vi "Create from Cluster.vi"(7 "Write Lock":refnum<notifier>, 8 "error in (no error)":errorcluster, 10 "Ref Data":T1={"Node Info"={"Index"=-1, "Parent"=-1, "Children"=[]}, "Owner"=refnum, "Changed"=FALSE, "Name"="", "Meta Data"=[], "Value Type"=enum."String", "Value"=variant}) -> (0 "error out":errorcluster, 3 "Config Element out":refnum<class "Config Element.lvclass">)   [LabVIEW 2023, in "CDM-Config.lvlib" / "Config Element.lvclass"]
uses:
  Config Element.lvclass
  Element Data.ctl
  Node Info.ctl
  Meta Data.ctl
  Value Type.ctl
  Config Element.lvclass/Config Element.ctl
  CDM-Config.lvlib
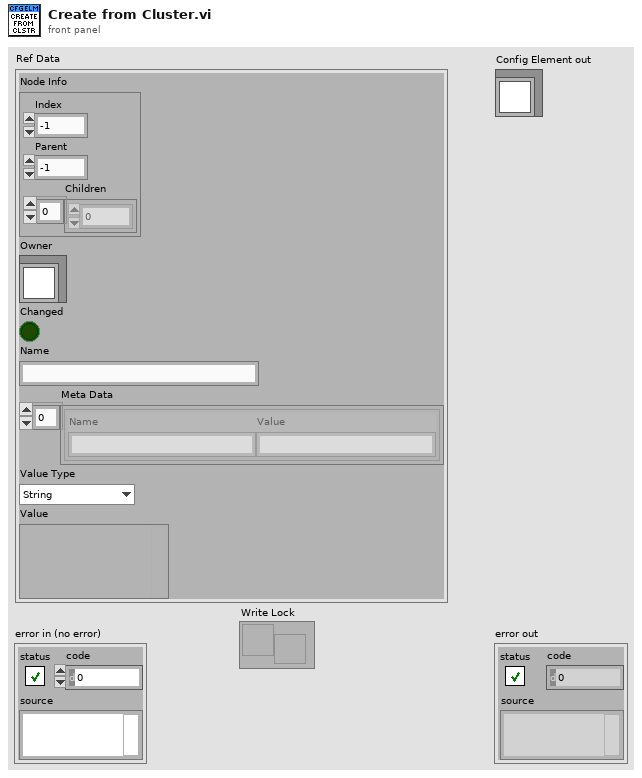
[diagram p1: front panel]
types:
  T1 = typedef "CDM-Config.lvlib/Config Element.lvclass/Element Data.ctl" = cluster{"Node Info":T2, "Owner":refnum<class>, "Changed":bool, "Name":string, "Meta Data":T3[], "Value Type":T4, "Value":variant}
  T2 = typedef "CDM-Config.lvlib/Node Info.ctl" = cluster{"Index":i32, "Parent":i32, "Children":i32[]}
  T3 = typedef "CDM-Config.lvlib/Meta Data.ctl" = cluster{"Name":string, "Value":string}
  T4 = typedef "CDM-Config.lvlib/Value Type.ctl" = enum16{"String", "Number", "Bool", "Object", "Array"}
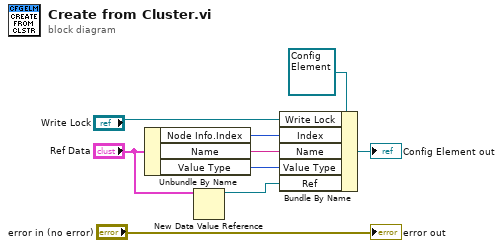
[diagram p0: block diagram]
diagram:
  n1 = Unbundle By Name("Ref Data") -> ("Node Info.Index"=w4:i32, "Name"=w3:string, "Value Type"=w2:T4)
  n2 = New Data Value Reference(data value="Ref Data") -> (data value reference=w6:refnum<data-value>)  [unwired: 1 in, 1 out]
  n3 = Bundle By Name(cluster=refnum<class "Config Element.lvclass"> refnum ("Config Element in"), "Write Lock"="Write Lock", "Index"=w4, "Name"=w3, "Value Type"=w2, "Ref"=w6) -> (→"Config Element out":refnum<class "Config Element.lvclass">)
  "error out" <- "error in (no error)"
